vi "GT Load Watch Fifo.vi"(8 "error in (no error)":errorcluster caption="错误输入（无错误）", 9 "pBuf":i16, 10 "fifo":i16, 11 "cardNum":i16) -> (0 "error out":errorcluster caption="错误输出", 1 "pBuf out":i16, 3 "function return":i16)   [LabVIEW 2020, in "gts1.lvlib"]
doc: "GT_API GT_LoadWatchFifo(short cardNum,short fifo,short *pBuf);"
uses:
  gts1.lvlib
  dll/32bit/multi_card/gts.dll
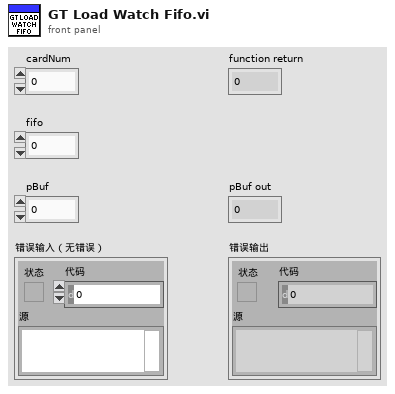
[diagram p1: front panel]
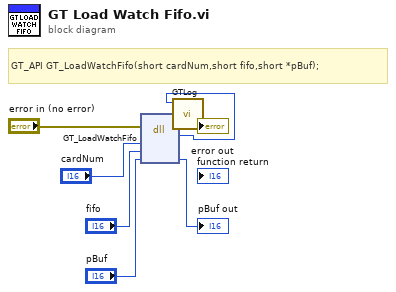
[diagram p0: block diagram]
diagram:
  # "GT_API GT_LoadWatchFifo(short cardNum,short fifo,short *pBuf);"
  n1 = dll-call lib="C:/1228/dll/32bit/multi_card/gts.dll" fn="GT_LoadWatchFifo"(error in="error in (no error)", "cardNum"="cardNum", "fifo"="fifo", "pBuf"="pBuf") -> (error out=w3:errorcluster, w1:i16, "pBuf"=→"pBuf out":i16)  [unwired: 4 in, 1 out]
  n2 = call "GTLog.vi"("error in (no error)"=w3, "Numeric"=w1) -> ("error out"=→"error out":errorcluster)  [unwired: 9 in]
